vi "GV-LightenLineColor.vi"(2 "Line color":u32(colorbox)) -> (6 "Light color":u32(colorbox))   [LabVIEW 2020, in "Sgraph_lib_V1.lvlib" / "Gviewer.lvclass"]
doc: "Andre Koelewijn, 30 june 2021\n\nLighten color for background min/max indication"
uses:
  Gviewer.lvclass
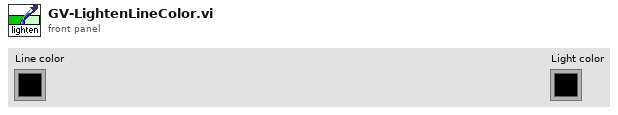
[diagram p1: front panel]
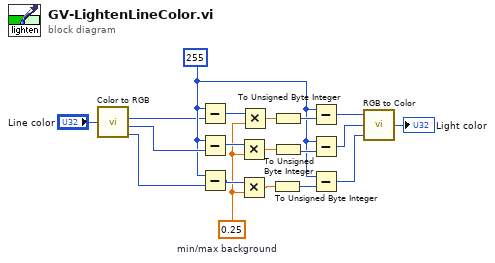
[diagram p0: block diagram]
diagram:
  w4 = u8 255 ("min/max background")
  w14 = 0.25  # min/max background
  n1 = call <vilib>:"Color to RGB.vi"("Color"="Line color") -> ("R"=w3:u8, "G"=w19:u8, "B"=w18:u8)  [unwired: 1 out]
  n2 = Subtract(x=w4, y=w3) -> (x-y=w15:u8)
  n3 = Subtract(x=w4, y=w19) -> (x-y=w16:u8)
  n4 = Subtract(x=w4, y=w18) -> (x-y=w17:u8)
  n5 = Multiply(x=w16, y=w14) -> (x*y=w12:dbl)
  n6 = Multiply(x=w17, y=w14) -> (x*y=w11:dbl)
  n7 = Multiply(x=w15, y=w14) -> (x*y=w13:dbl)
  n8 = To Unsigned Byte Integer(number=w11) -> (unsigned 8bit integer=w8:u8)
  n9 = To Unsigned Byte Integer(number=w13) -> (unsigned 8bit integer=w10:u8)
  n10 = To Unsigned Byte Integer(number=w12) -> (unsigned 8bit integer=w9:u8)
  n11 = Subtract(x=w4, y=w10) -> (x-y=w7:u8)
  n12 = Subtract(x=w4, y=w9) -> (x-y=w6:u8)
  n13 = Subtract(x=w4, y=w8) -> (x-y=w5:u8)
  n14 = call <vilib>:"RGB to Color.vi"("B"=w5, "G"=w6, "R"=w7) -> ("Color"=→"Light color":u32)
